vi "QC_MeasurementSetup.vi"() -> ()   [LabVIEW 2018]
uses:
  InstrControl/SupplyControl/SupplyControl.lvclass
  InstrControl/LCRControl/LCRControl.lvclass
  InstrControl/ProbeStationControl/ProbeStationControl.lvclass
  InstrControl/ArduinoControl/ArduinoControl.lvclass
  InstrControl/Switching/Switching.lvclass
  InstrControl/MultimeterControl/MultimeterControl.lvclass
panel:
  in  "GCD Measurement Parameters":T1={"Bias Supply"=refnum, "SMU"=refnum, "Arduino"=refnum, "Initial Voltage [V]"=-10.0, "Final Voltage [V]"=20.0, "Step Size [V]"=0.5, "Step Interval [s]"=1, "Number Of Steps"=51, "Ramp down steps [V]"=10.0, "Ramp down Interval [s]"=1, "Bias Voltage [V]"=5.0, "Set Current Limit?"=TRUE, "Current Limit [µA]"=1000.0, "Temperature Readout"=enum."Read Arduino", "Bias Supply Name"="Keithley 6517", "SMU Name"="Keithley 2410"} {"Current Limit [µA]" format="%.3f"; "Step Size [V]" format="%.1f"; "Final Voltage [V]" format="%.1f"; "Initial Voltage [V]" format="%.1f"}
  in  "Ris Measurement Parameters":T2={"Bias Supply"=refnum, "SMU"=refnum, "Multimeter"=refnum, "Arduino"=refnum, "Measurement switch"=refnum, "Initial Voltage [V]"=20.0, "Final Voltage [V]"=-500.0, "Step Size [V]"=20.0, "Step Interval [s]"=10, "Number Of Steps"=25, "Ramp down steps [V]"=10.0, "Ramp down Interval [s]"=1, "Set Current Limit?"=TRUE, "Current Limit [µA]"=1000.0, "Temperature Readout"=enum."Read Arduino", "Supply Name"="Keithley 487", "SMU Name"="Keithley 6517", "Voltmeter Name"="Keithley 2000", "R_is Limit [MOhm]"=-500.0, "Measurement switch used?"=FALSE, "Matrix X Channels"={"Bias Supply / SMU LO"=5, "Bias Supply / SMU HI"=6, "CV Box LO"=3, "CV Box HI"=4, "CV Box LO IN"=7, "CV Box HI IN"=8, "Volt meter LO"=1, "Volt meter HI"=2, "Mux1 C1"=9, "Mux1 C2"=10, "Mux2 C1"=11, "Mux2 C2"=12}} {"Current Limit [µA]" format="%.3f"; "Step Size [V]" format="%.1f"; "Final Voltage [V]" format="%.1f"; "Initial Voltage [V]" format="%.1f"}
  in  "Current Stability Measurement Parameters":T3={"Supply"=refnum, "DMM"=refnum, "DUT switch"=refnum, "Arduino"=refnum, "Measurement switch"=refnum, "Voltage [V]"=-700.0, "Measurement Interval [s]"=30, "Test Duration"=86400, "Ramp up steps [V]"=10.0, "Ramp up Interval [s]"=1, "Ramp down steps [V]"=10.0, "Ramp down Interval [s]"=1, "Set Current Limit?"=TRUE, "Current Limit [µA]"=1000.0, "Temperature Readout"=enum."Read Arduino", "Supply Name"="Keithley 2410", "DMM Name"="Keithley 2000", "Maximum current fluctuation [%]"=3.0, "Measurement switch used?"=FALSE, "DUT switch used?"=TRUE} {"Current Limit [µA]" format="%.3f"; "Test Duration" format="%<%H:%M:%S>t"; "Voltage [V]" format="%.1f"}
  in  "Cis Measurement Parameters":T4={"Supply"=refnum, "LCR"=refnum, "Arduino"=refnum, "Measurement switch"=refnum, "Initial Voltage [V]"=0.0, "Final Voltage [V]"=-500.0, "Step Size [V]"=10.0, "Step Interval [s]"=5, "Number Of Steps"=51, "AC frequency [Hz]"=100000, "RC Configuration"=1, "AC amplitude [V]"=0.1, "Ramp down steps [V]"=10.0, "Ramp down Interval [s]"=1, "Set Current Limit?"=TRUE, "Current Limit [µA]"=1000.0, "Temperature Readout"=enum."Read Arduino", "Supply Name"="Keithley 2410", "LCR Name"="WayneKerr 6440B", "C_is Limit [pF/cm]"=1.0, "Measurement switch used?"=FALSE} {"Current Limit [µA]" format="%.3f"; "RC Configuration" items=["serial", "parallel"]; "Step Size [V]" format="%.1f"; "Final Voltage [V]" format="%.1f"; "Initial Voltage [V]" format="%.1f"}
  in  "CV Measurement Parameters":T5={"Supply"=refnum, "LCR"=refnum, "Arduino"=refnum, "Measurement switch"=refnum, "Initial Voltage [V]"=0.0, "Final Voltage [V]"=-500.0, "Step Size [V]"=10.0, "Step Interval [s]"=10, "Number Of Steps"=51, "Ramp down steps [V]"=10.0, "Ramp down Interval [s]"=1, "Set Current Limit?"=TRUE, "Current Limit [µA]"=1.0, "Temperature Readout"=enum."Read Arduino", "Supply Name"="Keithley 237", "LCR Name"="HP 4284A", "V_depletion Limit [V]"=-300.0, "Measurement switch used?"=FALSE} {"Current Limit [µA]" format="%.3f"; "Step Size [V]" format="%.1f"; "Final Voltage [V]" format="%.1f"; "Initial Voltage [V]" format="%.1f"}
  in  "IV Measurement Parameters":T6={"Supply"=refnum, "Arduino"=refnum, "Measurement switch"=refnum, "Initial Voltage [V]"=0.0, "Final Voltage [V]"=-700.0, "Step Size [V]"=10.0, "Step Interval [s]"=10, "Number Of Steps"=71, "Ramp down steps [V]"=10.0, "Ramp down Interval [s]"=1, "hold steps"=3, "Set Current Limit?"=TRUE, "Current Limit [µA]"=1.0, "Temperature Readout"=enum."Read Arduino", "Supply Name"="Keithley 237", "V_breakdown Limit [V]"=-500.0, "Measurement switch used?"=FALSE} {"Current Limit [µA]" format="%.3f"; "Step Size [V]" format="%.1f"; "Final Voltage [V]" format="%.1f"; "Initial Voltage [V]" format="%.1f"}
  in  "Striptest Measurement Parameters":T7={"Bias Supply"=refnum, "SMU"=refnum, "LCR"=refnum, "ProbeStation"=refnum, "Arduino"=refnum, "Measurement switch"=refnum, "Probe Card Channels"=1, "Bias Voltage [V]"=-350.0, "First strip"=1, "Last strip"=1280, "Base Voltage [V]"=10.0, "Base Ramp Step [V]"=10.0, "Base Ramp Interval [ms]"=1000, "High Voltage [V]"=100.0, "High Ramp Step [V]"=100.0, "High Ramp Interval [ms]"=1000, "AC frequency [Hz]"=1000, "AC amplitude [V]"=0.1, "RC Configuration"=0, "Single Needle"=FALSE, "Temperature Readout"=enum."Read Arduino", "Fraction of good strips [%]"=98.0, "Measurement switch used?"=FALSE, "Matrix X Channels"={"Mux1 C1"=9, "Mux1 C2"=10, "Mux2 C1"=11, "Mux2 C2"=12}, "Pinholes Y/N"=TRUE, "Capacitance Y/N"=TRUE, "Resistance Y/N"=TRUE, "Bias Supply Name"="Keithley 6517", "SMU Name"="Keithley 2410", "LCR Name"="Wayne Kerr 6440B"} {"RC Configuration" items=["serial", "parallel"]; "High Ramp Step [V]" format="%.1f"; "High Voltage [V]" format="%.1f"; "Base Ramp Step [V]" format="%.1f"; "Base Voltage [V]" format="%.1f"; "Bias Voltage [V]" format="%.1f"}
  # "Main Sensor Tests"
  # "Halfmoon-exclusive Tests"
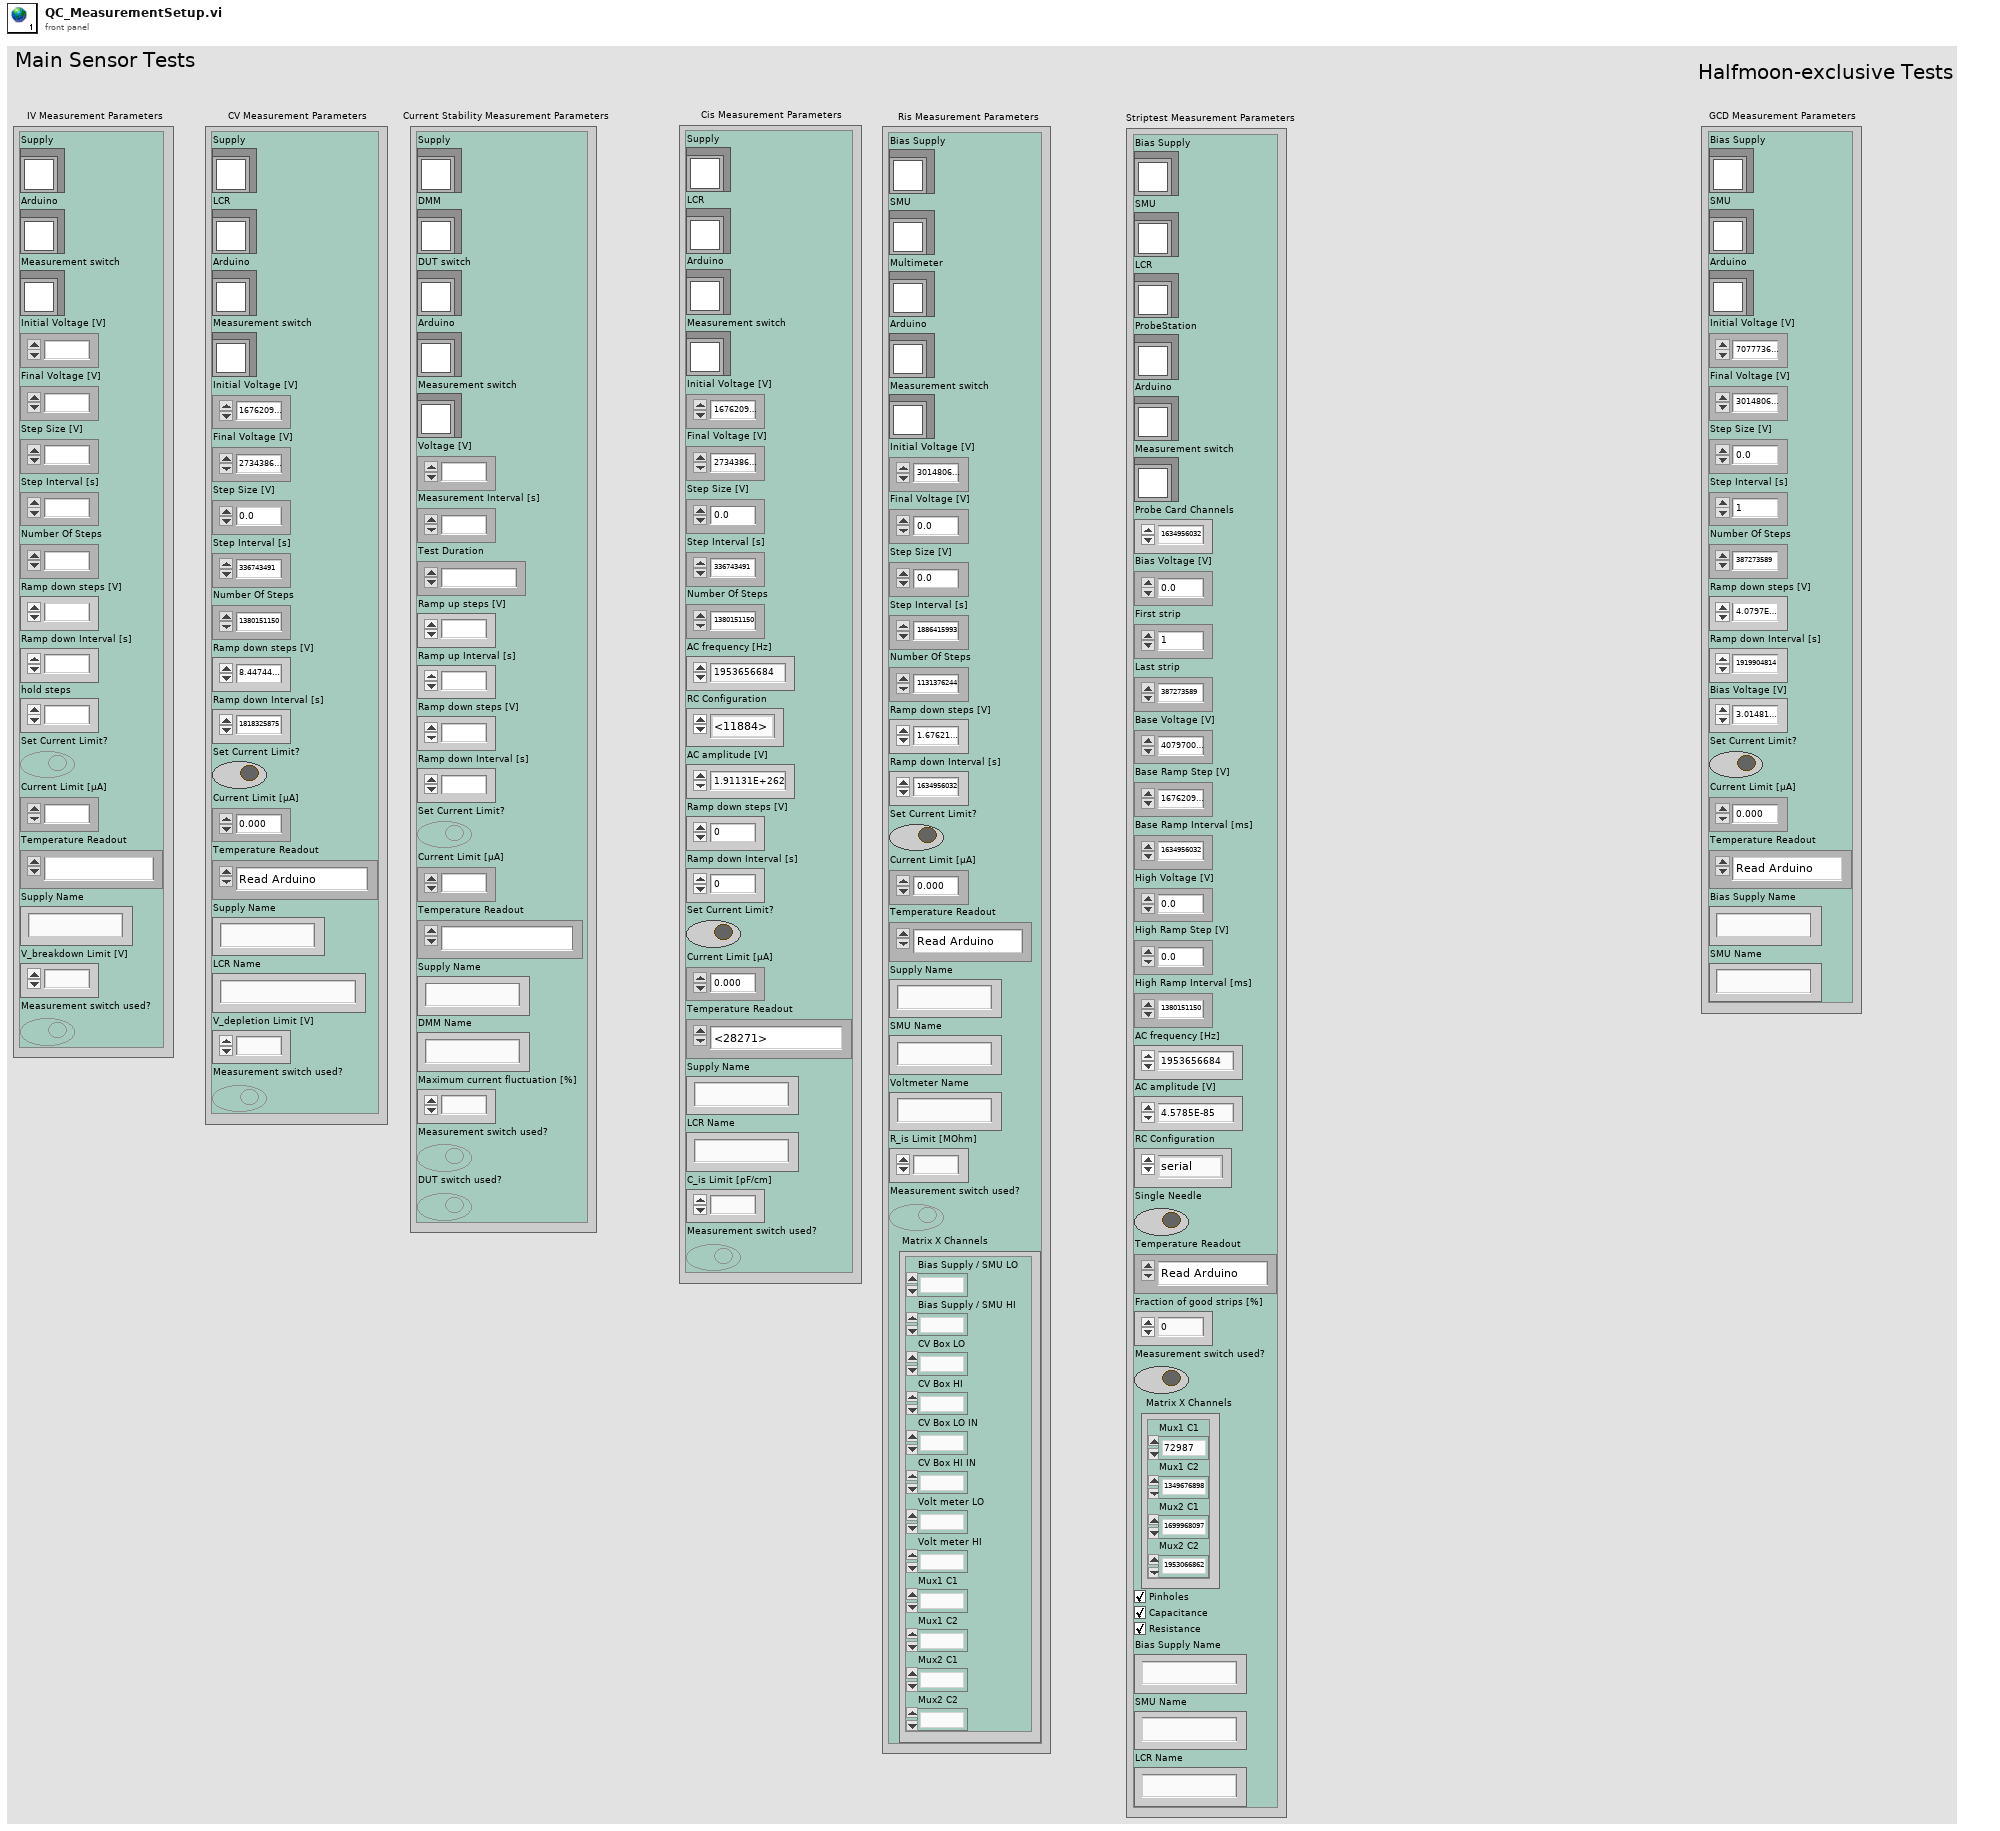
[diagram p1: front panel]
types:
  T1 = cluster{"Bias Supply":refnum<class "SupplyControl.lvclass">, "SMU":refnum<class "SupplyControl.lvclass">, "Arduino":refnum<class "ArduinoControl.lvclass">, "Initial Voltage [V]":dbl, "Final Voltage [V]":dbl, "Step Size [V]":dbl, "Step Interval [s]":i32, "Number Of Steps":u32, "Ramp down steps [V]":dbl, "Ramp down Interval [s]":i32, "Bias Voltage [V]":dbl, "Set Current Limit?":bool, "Current Limit [µA]":dbl, "Temperature Readout":enum16{"Read Arduino", "Enter manually"}, "Bias Supply Name":string, "SMU Name":string}
  T2 = cluster{"Bias Supply":refnum<class "SupplyControl.lvclass">, "SMU":refnum<class "SupplyControl.lvclass">, "Multimeter":refnum<class "MultimeterControl.lvclass">, "Arduino":refnum<class "ArduinoControl.lvclass">, "Measurement switch":refnum<class "Switching.lvclass">, "Initial Voltage [V]":dbl, "Final Voltage [V]":dbl, "Step Size [V]":dbl, "Step Interval [s]":i32, "Number Of Steps":u32, "Ramp down steps [V]":dbl, "Ramp down Interval [s]":i32, "Set Current Limit?":bool, "Current Limit [µA]":dbl, "Temperature Readout":enum16{"Read Arduino", "Enter manually"}, "Supply Name":string, "SMU Name":string, "Voltmeter Name":string, "R_is Limit [MOhm]":dbl, "Measurement switch used?":bool, "Matrix X Channels":cluster{"Bias Supply / SMU LO":i32, "Bias Supply / SMU HI":i32, "CV Box LO":i32, "CV Box HI":i32, "CV Box LO IN":i32, "CV Box HI IN":i32, "Volt meter LO":i32, "Volt meter HI":i32, "Mux1 C1":i32, "Mux1 C2":i32, "Mux2 C1":i32, "Mux2 C2":i32}}
  T3 = cluster{"Supply":refnum<class "SupplyControl.lvclass">, "DMM":refnum<class "MultimeterControl.lvclass">, "DUT switch":refnum<class "Switching.lvclass">, "Arduino":refnum<class "ArduinoControl.lvclass">, "Measurement switch":refnum<class "Switching.lvclass">, "Voltage [V]":dbl, "Measurement Interval [s]":i32, "Test Duration":u32, "Ramp up steps [V]":dbl, "Ramp up Interval [s]":u32, "Ramp down steps [V]":dbl, "Ramp down Interval [s]":i32, "Set Current Limit?":bool, "Current Limit [µA]":dbl, "Temperature Readout":enum16{"Read Arduino", "Enter manually"}, "Supply Name":string, "DMM Name":string, "Maximum current fluctuation [%]":dbl, "Measurement switch used?":bool, "DUT switch used?":bool}
  T4 = cluster{"Supply":refnum<class "SupplyControl.lvclass">, "LCR":refnum<class "LCRControl.lvclass">, "Arduino":refnum<class "ArduinoControl.lvclass">, "Measurement switch":refnum<class "Switching.lvclass">, "Initial Voltage [V]":dbl, "Final Voltage [V]":dbl, "Step Size [V]":dbl, "Step Interval [s]":i32, "Number Of Steps":u32, "AC frequency [Hz]":i32, "RC Configuration":u16, "AC amplitude [V]":dbl, "Ramp down steps [V]":dbl, "Ramp down Interval [s]":i32, "Set Current Limit?":bool, "Current Limit [µA]":dbl, "Temperature Readout":enum16{"Read Arduino", "Enter manually"}, "Supply Name":string, "LCR Name":string, "C_is Limit [pF/cm]":dbl, "Measurement switch used?":bool}
  T5 = cluster{"Supply":refnum<class "SupplyControl.lvclass">, "LCR":refnum<class "LCRControl.lvclass">, "Arduino":refnum<class "ArduinoControl.lvclass">, "Measurement switch":refnum<class "Switching.lvclass">, "Initial Voltage [V]":dbl, "Final Voltage [V]":dbl, "Step Size [V]":dbl, "Step Interval [s]":i32, "Number Of Steps":u32, "Ramp down steps [V]":dbl, "Ramp down Interval [s]":i32, "Set Current Limit?":bool, "Current Limit [µA]":dbl, "Temperature Readout":enum16{"Read Arduino", "Enter manually"}, "Supply Name":string, "LCR Name":string, "V_depletion Limit [V]":dbl, "Measurement switch used?":bool}
  T6 = cluster{"Supply":refnum<class "SupplyControl.lvclass">, "Arduino":refnum<class "ArduinoControl.lvclass">, "Measurement switch":refnum<class "Switching.lvclass">, "Initial Voltage [V]":dbl, "Final Voltage [V]":dbl, "Step Size [V]":dbl, "Step Interval [s]":i32, "Number Of Steps":u32, "Ramp down steps [V]":dbl, "Ramp down Interval [s]":i32, "hold steps":i32, "Set Current Limit?":bool, "Current Limit [µA]":dbl, "Temperature Readout":enum16{"Read Arduino", "Enter manually"}, "Supply Name":string, "V_breakdown Limit [V]":dbl, "Measurement switch used?":bool}
  T7 = cluster{"Bias Supply":refnum<class "SupplyControl.lvclass">, "SMU":refnum<class "SupplyControl.lvclass">, "LCR":refnum<class "LCRControl.lvclass">, "ProbeStation":refnum<class "ProbeStationControl.lvclass">, "Arduino":refnum<class "ArduinoControl.lvclass">, "Measurement switch":refnum<class "Switching.lvclass">, "Probe Card Channels":i32, "Bias Voltage [V]":dbl, "First strip":i32, "Last strip":i32, "Base Voltage [V]":dbl, "Base Ramp Step [V]":dbl, "Base Ramp Interval [ms]":u32, "High Voltage [V]":dbl, "High Ramp Step [V]":dbl, "High Ramp Interval [ms]":u32, "AC frequency [Hz]":i32, "AC amplitude [V]":dbl, "RC Configuration":u16, "Single Needle":bool, "Temperature Readout":enum16{"Read Arduino", "Enter manually"}, "Fraction of good strips [%]":dbl, "Measurement switch used?":bool, "Matrix X Channels":cluster{"Mux1 C1":i32, "Mux1 C2":i32, "Mux2 C1":i32, "Mux2 C2":i32}, "Pinholes Y/N":bool, "Capacitance Y/N":bool, "Resistance Y/N":bool, "Bias Supply Name":string, "SMU Name":string, "LCR Name":string}
diagram:
